vi "one_button_dialog_hello_world.vi"   [LabVIEW 2021]
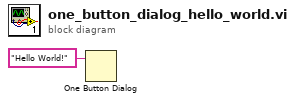
[diagram p0: block diagram]
diagram:
  n1 = One Button Dialog(message="Hello World!") -> ()  [unwired: 1 in, 1 out]
